vi "Pneumatics_Command_Set.vi"   [LabVIEW 2016]
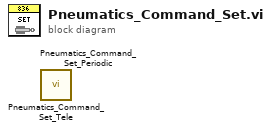
[diagram p0: block diagram]
diagram:
  n1 = call <userlib>:"Pneumatics_Command_Set_Tele.vi"() -> ()  [unwired: 11 in, 1 out]
  n2 = call <userlib>:"Pneumatics_Command_Set_Periodic.vi"() -> ()  [unwired: 11 in, 1 out]
